vi "Keithley 24XX Read Single.vi"() -> ()   [LabVIEW 2021]
doc: "This example shows how to configure a measurement and take a reading."
uses:
  <instrlib>/Keithley 24XX/Public/Data/Read (Single Point).vi
  <instrlib>/Keithley 24XX/Keithley 24XX.lvlib
panel:
  in  "Vin SMU":refnum<visa-resource-name>
  out "Vin SMU Voltage":sgl
  out "Vin SMU Current":sgl
  in  "Vin SMU Voltage Manual Range":dbl=1.0
  in  "Vin SMU Current Manual Range":dbl=1.0
  in  "Vin SMU Resistance Manual Range":dbl=1.0
  in  "Vin SMU Output Level":dbl
  in  "Vin SMU Compliance  Leve":dbl=0.1
  in  "Vin SMU Source Mode":u16(ring) items=["Voltage", "Current"]
  in  "error in":errorcluster
  out "error out":errorcluster
  in  "Load SMU Source Mode":u16(ring) items=["Voltage", "Current"]
  in  "Load SMU Compliance  Level (0.1)":dbl=0.1
  in  "Load SMU Output Level (0)":dbl
  in  "Load SMU Resistance Manual Range":dbl=1.0
  in  "Load SMU Current Manual Range":dbl=1.0
  in  "Load SMU Voltage Manual Range":dbl=1.0
  out "Load SMU Current":sgl
  out "Load SMU Voltage":sgl
  in  "Load SMU":refnum<visa-resource-name>
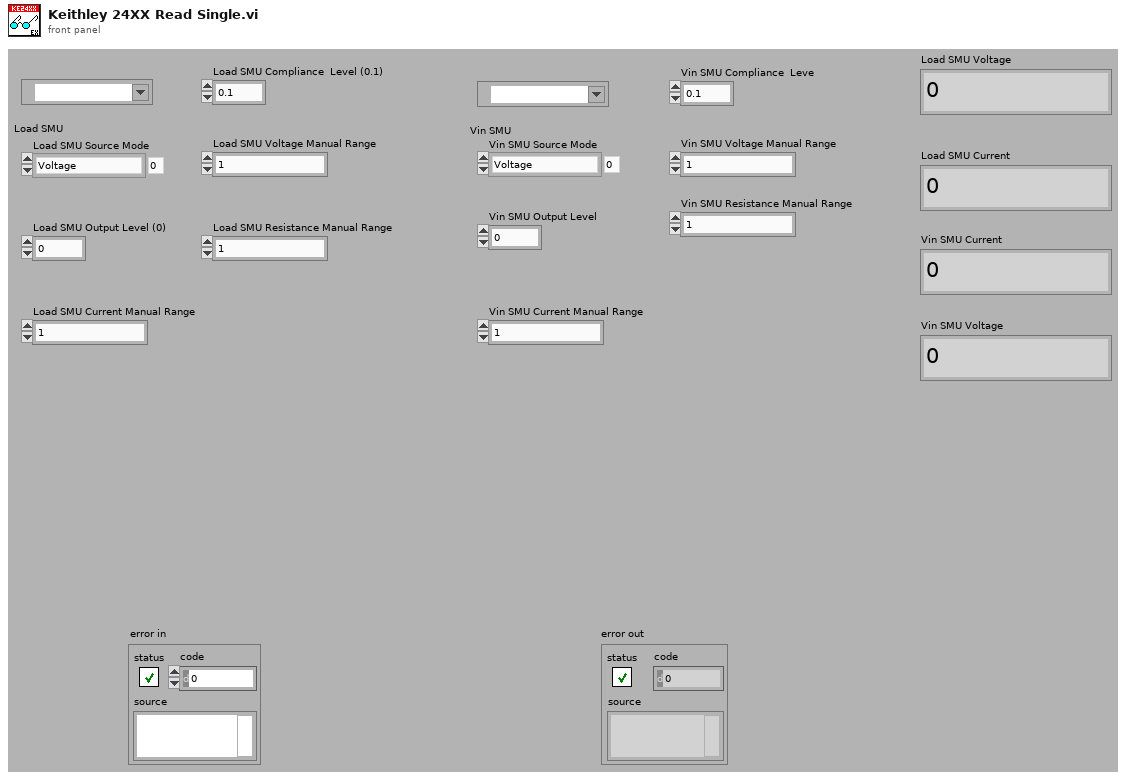
[diagram p1: front panel]
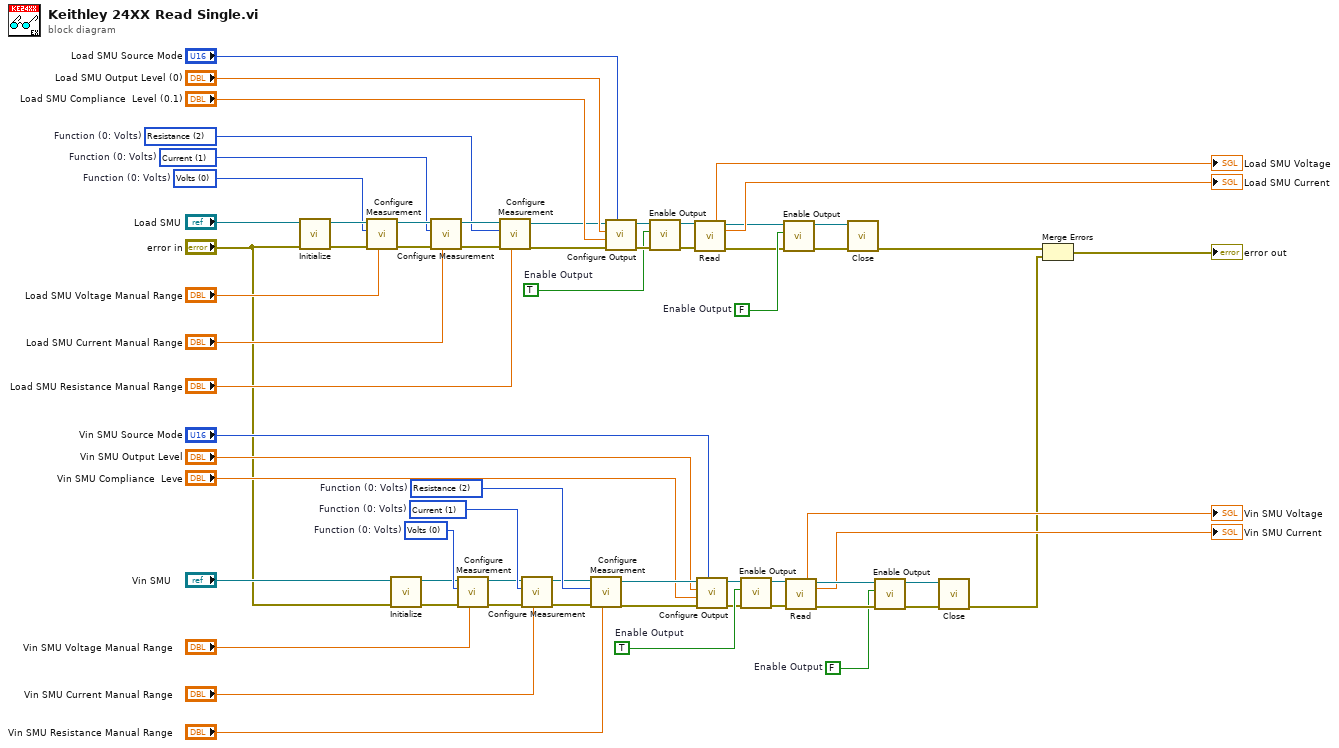
[diagram p0: block diagram]
diagram:
  w30 = TRUE  # Enable Output
  w19 = FALSE  # Enable Output
  w15 = u16 2 items=["Volts", "Current", "Resistance"]  # Function (0: Volts)
  w14 = u16 1 items=["Volts", "Current", "Resistance"]  # Function (0: Volts)
  w13 = u16 0 items=["Volts", "Current", "Resistance"]  # Function (0: Volts)
  w38 = TRUE  # Enable Output
  w49 = FALSE  # Enable Output
  w53 = u16 2 items=["Volts", "Current", "Resistance"]  # Function (0: Volts)
  w54 = u16 1 items=["Volts", "Current", "Resistance"]  # Function (0: Volts)
  w55 = u16 0 items=["Volts", "Current", "Resistance"]  # Function (0: Volts)
  n1 = call <instrlib>:"Initialize.vi"("error in (no error)"="error in", "VISA resource name"="Load SMU") -> ("error out"=w60:errorcluster, "VISA resource name out"=w61:refnum<visa-resource-name>)  [unwired: 8 in]
  n2 = call <instrlib>:"Configure Measurement.vi"("Manual Range (1.0)"="Load SMU Voltage Manual Range", "error in (no error)"=w60, "Function (0: Volts)"=w55, "VISA resource name"=w61) -> ("error out"=w58:errorcluster, "VISA resource name out"=w59:refnum<visa-resource-name>)  [unwired: 6 in]
  n3 = call <instrlib>:"Initialize.vi"("error in (no error)"="error in", "VISA resource name"="Vin SMU") -> ("error out"=w8:errorcluster, "VISA resource name out"=w7:refnum<visa-resource-name>)  [unwired: 8 in]
  n4 = call <instrlib>:"Configure Measurement.vi"("Manual Range (1.0)"="Load SMU Current Manual Range", "error in (no error)"=w58, "Function (0: Volts)"=w54, "VISA resource name"=w59) -> ("error out"=w57:errorcluster, "VISA resource name out"=w56:refnum<visa-resource-name>)  [unwired: 6 in]
  n5 = call <instrlib>:"Configure Measurement.vi"("Manual Range (1.0)"="Vin SMU Voltage Manual Range", "error in (no error)"=w8, "Function (0: Volts)"=w13, "VISA resource name"=w7) -> ("error out"=w10:errorcluster, "VISA resource name out"=w9:refnum<visa-resource-name>)  [unwired: 6 in]
  n6 = call <instrlib>:"Configure Measurement.vi"("Manual Range (1.0)"="Load SMU Resistance Manual Range", "error in (no error)"=w57, "Function (0: Volts)"=w53, "VISA resource name"=w56) -> ("error out"=w37:errorcluster, "VISA resource name out"=w36:refnum<visa-resource-name>)  [unwired: 6 in]
  n7 = call <instrlib>:"Configure Measurement.vi"("Manual Range (1.0)"="Vin SMU Current Manual Range", "error in (no error)"=w10, "Function (0: Volts)"=w14, "VISA resource name"=w9) -> ("error out"=w11:errorcluster, "VISA resource name out"=w12:refnum<visa-resource-name>)  [unwired: 6 in]
  n8 = call <instrlib>:"Configure Measurement.vi"("Manual Range (1.0)"="Vin SMU Resistance Manual Range", "error in (no error)"=w11, "Function (0: Volts)"=w15, "VISA resource name"=w12) -> ("error out"=w31:errorcluster, "VISA resource name out"=w32:refnum<visa-resource-name>)  [unwired: 6 in]
  n9 = call <instrlib>:"Configure Output.vi"("Source Mode  (0: Voltage)"="Load SMU Source Mode", "error in (no error)"=w37, "Compliance  Level (0.1)"="Load SMU Compliance  Level (0.1)", "Output Level (0)"="Load SMU Output Level (0)", "VISA resource name"=w36) -> ("error out"=w39:errorcluster, "VISA resource name out"=w40:refnum<visa-resource-name>)  [unwired: 5 in]
  n10 = call <instrlib>:"Enable Output.vi"("error in (no error)"=w39, "Enable Output (T: Enable)"=w38, "VISA resource name"=w40) -> ("error out"=w42:errorcluster, "VISA resource name out"=w41:refnum<visa-resource-name>)  [unwired: 7 in]
  n11 = call-poly <instrlib>:"Read.vi"("VISA resource name"=w41, "error in (no error)"=w42) -> ("Voltage"=→"Load SMU Voltage":sgl, "VISA resource name out"=w43:refnum<visa-resource-name>, "Current"=→"Load SMU Current":sgl, "error out"=w44:errorcluster)  [unwired: 7 in, 3 out]
  n12 = call <instrlib>:"Configure Output.vi"("Source Mode  (0: Voltage)"="Vin SMU Source Mode", "error in (no error)"=w31, "Compliance  Level (0.1)"="Vin SMU Compliance  Leve", "Output Level (0)"="Vin SMU Output Level", "VISA resource name"=w32) -> ("error out"=w29:errorcluster, "VISA resource name out"=w28:refnum<visa-resource-name>)  [unwired: 5 in]
  n13 = call <instrlib>:"Enable Output.vi"("error in (no error)"=w29, "Enable Output (T: Enable)"=w30, "VISA resource name"=w28) -> ("error out"=w26:errorcluster, "VISA resource name out"=w27:refnum<visa-resource-name>)  [unwired: 7 in]
  n14 = call <instrlib>:"Enable Output.vi"("error in (no error)"=w44, "Enable Output (T: Enable)"=w49, "VISA resource name"=w43) -> ("error out"=w45:errorcluster, "VISA resource name out"=w46:refnum<visa-resource-name>)  [unwired: 7 in]
  n15 = call-poly <instrlib>:"Read.vi"("VISA resource name"=w27, "error in (no error)"=w26) -> ("Voltage"=→"Vin SMU Voltage":sgl, "VISA resource name out"=w25:refnum<visa-resource-name>, "Current"=→"Vin SMU Current":sgl, "error out"=w24:errorcluster)  [unwired: 7 in, 3 out]
  n16 = call <instrlib>:"Close.vi"("error in (no error)"=w45, "VISA resource name"=w46) -> ("error out"=w34:errorcluster)  [unwired: 9 in]
  n17 = call <instrlib>:"Enable Output.vi"("error in (no error)"=w24, "Enable Output (T: Enable)"=w19, "VISA resource name"=w25) -> ("error out"=w23:errorcluster, "VISA resource name out"=w22:refnum<visa-resource-name>)  [unwired: 7 in]
  n18 = call <instrlib>:"Close.vi"("error in (no error)"=w23, "VISA resource name"=w22) -> ("error out"=w1:errorcluster)  [unwired: 9 in]
  n19 = Merge Errors(w34, w1) -> (→"error out":errorcluster)
